vi "UDP Rx Main.vi"(8 "error in (no error)":errorcluster, 9 "max size (800)":i32=800, 10 "ports":u16[](array[numeric])=[60000, 60001, 60002, 60003], 11 "Stop Pointer":refnum<class "Pointer.lvclass">) -> (0 "error out":errorcluster)   [LabVIEW 2017]
uses:
  <vilib>/NI/Memory Manager/Classes/Pointer/Pointer.lvclass
  <vilib>/NI/Memory Manager/Classes/Pointer/Pointer.lvclass/Pointer.ctl
  <vilib>/NI/Memory Manager/Classes/Pointer/Write Bool.vi
  <vilib>/NI/Memory Manager/Classes/Pointer/Read I32.vi
  <vilib>/NI/Memory Manager/Classes/Pointer/Read Bool.vi
  <vilib>/NI/Memory Manager/Classes/Pointer/Get Address.vi
  <vilib>/NI/Memory Manager/Classes/Pointer/Set Address.vi
  <vilib>/NI/Memory Manager/Classes/Pointer/Set Size.vi
  <vilib>/NI/Memory Manager/Classes/Pointer/Set Internal.vi
  <vilib>/NI/Memory Manager/Classes/Pointer/Clear.vi
  <vilib>/NI/Memory Manager/Classes/Pointer/Write (No Check).vi
  <vilib>/NI/Memory Manager/Classes/Pointer/Write (No Check) Bool.vi
  <vilib>/NI/Memory Manager/Classes/Pointer/Check Move.vi
  <vilib>/NI/Memory Manager/Classes/Pointer/Read (No Check).vi
  <vilib>/NI/Memory Manager/Classes/Pointer/Read (No Check) I32.vi
  <vilib>/NI/Memory Manager/Classes/Pointer/Read (No Check) Bool.vi
  <vilib>/NI/Memory Manager/Classes/Pointer/Check Null Pointer.vi
  <vilib>/NI/Memory Manager/Classes/Pointer/Clear (No Check).vi
  <vilib>/NI/Memory Manager/Classes/Pointer/Check Length.vi
  <vilib>/NI/Memory Manager/Classes/Pointer/Check Count.vi
  <vilib>/NI/Memory Manager/Classes/Pointer/Check Bounds (Power of 2).vi
  <vilib>/NI/Memory Manager/Classes/Pointer/Errors.vi
  <vilib>/NI/Memory Manager/Classes/Pointer/Null Pointer.vi
  <vilib>/NI/Memory Manager/Classes/Pointer/Get Size.vi
  <vilib>/NI/Memory Manager/Classes/Pointer/Check Bounds (Pointer).vi
  <vilib>/NI/Memory Manager/Classes/Pointer/Out of Bounds.vi
  <vilib>/NI/Memory Manager/Classes/Pointer/Check Bounds.vi
  <vilib>/NI/Memory Manager/Classes/Pointer/Create Error.vi
  <vilib>/NI/Memory Manager/Classes/Pointer/Write Pointer Size to Error.vi
  <vilib>/NI/Memory Manager/Classes/Pointer/Check Bounds (Buffer).vi
  <vilib>/NI/Memory Manager/Constants/Constants.vi
  <vilib>/NI/Memory Manager/Constants/Library Name.vi
  <vilib>/NI/Memory Manager/Classes/Pointer/Pointer Error Info.vi
  <vilib>/NI/Memory Manager/Constants/Pointer Class Name.vi
  <vilib>/NI/Memory Manager/Classes/Pointer/Buffer Underflow.vi
  <vilib>/NI/Memory Manager/VIs/New Error Cluster.vi
  <vilib>/NI/Memory Manager/VIs/New Error Cluster (512B).vi
  <vilib>/NI/Memory Manager/VIs/Set Error Status.vi
  <vilib>/NI/Memory Manager/VIs/Set Error Code.vi
  <vilib>/NI/Memory Manager/VIs/Set Error Source.vi
  <vilib>/NI/Memory Manager/VIs/Write String to Source.vi
  <vilib>/NI/Memory Manager/VIs/Write Numeric to Source.vi
  <vilib>/NI/Memory Manager/VIs/Write Numeric Scalar to Source (Base10 U64).vi
panel:
  out "rx counts":i32[](array[numeric])
  in  "Stop":bool
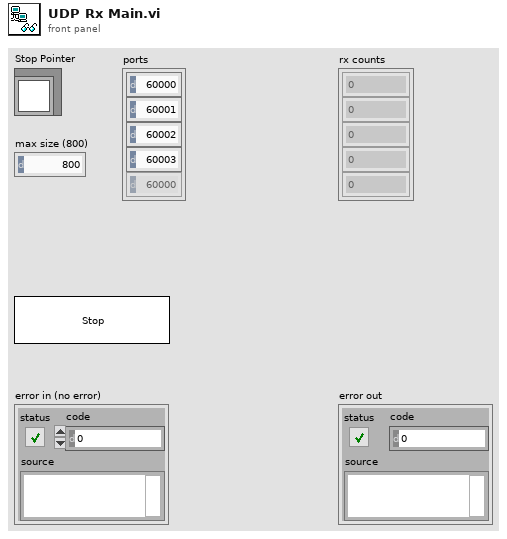
[diagram p1: front panel]
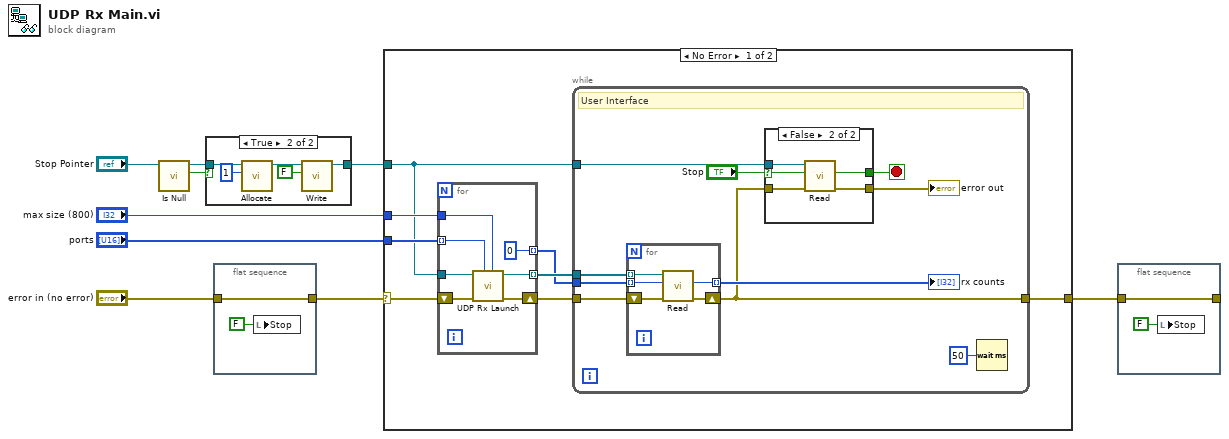
[diagram p0: block diagram]
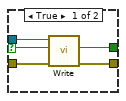
[diagram p3: hidden frame]
diagram:
  n1 = call <vilib>:"Is Null.vi"("Pointer in"="Stop Pointer") -> ("null?"=w1:bool, "Pointer out"=w2:refnum<class "Pointer.lvclass">)  [unwired: 8 in, 1 out]
  n2 = case shown="True" w1 {
    tunnel: [w10 w13] -> w4
    tunnel: w2 -> [w10 w11]
    frame False {
    }
    frame True {
      n3 = call <vilib>:"Allocate.vi"("size"=u64 1, "Pointer type"=w11) -> ("Pointer out"=w14:refnum<class "Pointer.lvclass">)  [unwired: 8 in, 1 out]
      n4 = call-poly <vilib>:"Write.vi"("value"=FALSE, "Pointer in"=w14) -> ("Pointer out"=w13:refnum<class "Pointer.lvclass">)  [unwired: 6 in, 3 out]
    }
  }
  n5 = flat-sequence {
    tunnel: "error in (no error)" -> [w17]
    tunnel: [w17] -> w5
    frame #0 {
      n6 = local write "Stop"(FALSE ("Stop")) -> ()
    }
  }
  n7 = case shown="No Error" w5 {
    selector: w5 -> [w19 w58]
    tunnel: "ports" -> [w25 _]
    tunnel: "max size (800)" -> [w24 _]
    tunnel: w4 -> [w21 _]
    tunnel: [w20 w58] -> w6
    frame No Error {
      n8 = for {
        tunnel: w21 -> [w27]
        tunnel: w25 -> [w30] mode=indexing
        tunnel: w24 -> [w29]
        shift-right: [w32] -> w23
        shift-left: w19 -> [w31]
        tunnel: [w28] -> w22 mode=indexing
        tunnel: [0] -> w18 mode=indexing
        n9 = call "UDP Rx Launch.vi"("max size (548)"=w29, "port"=w30, "error in (no error)"=w31, "Stop Pointer"=w27) -> ("error out"=w32:errorcluster, "Count Pointer"=w28:refnum<class "Pointer.lvclass">)  [unwired: 6 in]
      }
      n10 = while {
        tunnel: w23 -> [w41]
        tunnel: w22 -> [w42]
        tunnel: w21 -> [w40]
        tunnel: [w34] -> w20
        tunnel: w18 -> [w33]
        stop <- w39 stop-if-true
        # "User Interface"
        n11 = for {
          tunnel: w42 -> [w57] mode=indexing
          tunnel: [w54] -> w36 mode=indexing
          shift-right: [w55] -> w34
          shift-left: w41 -> [w56]
          tunnel: w33 -> [w53] mode=indexing
          n12 = call-poly <vilib>:"Read.vi"("error in (no error)"=w56, "value in"=w53, "Pointer in"=w57) -> ("error out"=w55:errorcluster, "value out"=w54:i32)  [unwired: 5 in, 2 out]
        }
        "rx counts" <- w36
        n13 = case shown="False" "Stop" {
          selector: "Stop" -> [w43 w48]
          tunnel: w40 -> [w47 w52]
          tunnel: w34 -> [w46 w51]
          tunnel: [w45 w50] -> w39
          tunnel: [w44 w49] -> w37
          frame True {
            n14 = call-poly <vilib>:"Write.vi"("error in (no error)"=w46, "value"=w43, "Pointer in"=w47) -> ("error out"=w44:errorcluster, "value"=w45:bool)  [unwired: 5 in, 2 out]
          }
          frame False {
            n15 = call-poly <vilib>:"Read.vi"("error in (no error)"=w51, "value in"=w48, "Pointer in"=w52) -> ("error out"=w49:errorcluster, "value out"=w50:bool)  [unwired: 5 in, 2 out]
          }
        }
        "error out" <- w37
        n16 = Wait (ms)(milliseconds to wait=u32 50) -> ()  [unwired: 1 out]
      }
    }
    frame Error {
    }
  }
  n17 = flat-sequence {
    tunnel: w6 -> [w60]
    tunnel: [w60] -> _
    frame #0 {
      n18 = local write "Stop"(FALSE ("Stop")) -> ()
    }
  }
